vi "arrayU8.vi"(2 "Array In":u8[](array[numeric]), 3 "Base":u8) -> (0 "Array out (not inplace)":u8[](array[numeric]), 1 "Array Out":u8[](array[numeric]))   [LabVIEW 2013]
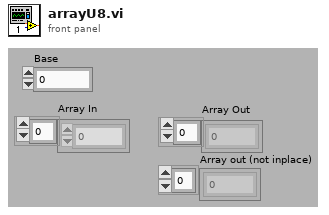
[diagram p1: front panel]
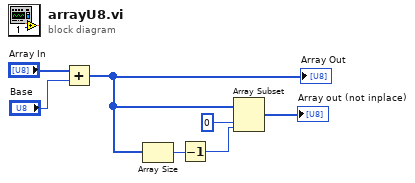
[diagram p0: block diagram]
diagram:
  n1 = Add(x="Array In", y="Base") -> (x+y=w2:u8[])
  "Array Out" <- w2
  n2 = Array Size(array=w2) -> (size(s)=w5:i32)
  n3 = Decrement(x=w5) -> (x-1=w6:i32)
  n4 = Array Subset(array=w2, index=0, length=w6) -> (→"Array out (not inplace)":u8[])
